vi "Tacking Helper - Waypoint Array Constructor.vi"(0 "Second Angle":dbl, 1 "Minimum Final Tack Distance (m?)":dbl, 2 "Starting\nArm Length":dbl, 3 "Second\nArm Length":dbl, 5 "Jump Length (m)":dbl, 7 "Starting Angle":dbl, 9 "Distance of each waypoint to boat":dbl[](array[numeric]), 12 "Array Beginning":i32, 13 "Waypoint Array In":T1[](array[typedef]), 14 "Boat Position":T3) -> (4 "Distance to boat":dbl, 6 "Final Index of\nWaypoint Array":i32, 8 "Intermediate \nWaypoint Array out":T1[](array[typedef]))   [LabVIEW 2011]
doc: "While the distance to the boat is greater than 1 jump (plus a minimum tack distance allowable we have yet to determine) the while loop will increment again and another two points will be calculated (one jump). The subvi inside of the loop takes the angles and lengths and actually adds the next step to the array.\n\nThe intermediate waypoint array output is the important thing - it stores each waypoint. The 'final index' and 'distance until boat' are used for plotting."
uses:
  2 Typedefs/UTM Location.ctl
  0x2-OCU-Think Comm/0x2 Typedefs/ocuWaypoint.ctl
  0x2-OCU-Think Comm/0x2 Typedefs/waypointTypes.ctl
  <vilib>/Analysis/_algsub.llb/Real Vector Norm.vi
  <vilib>/Analysis/NI_AALPro.lvlib
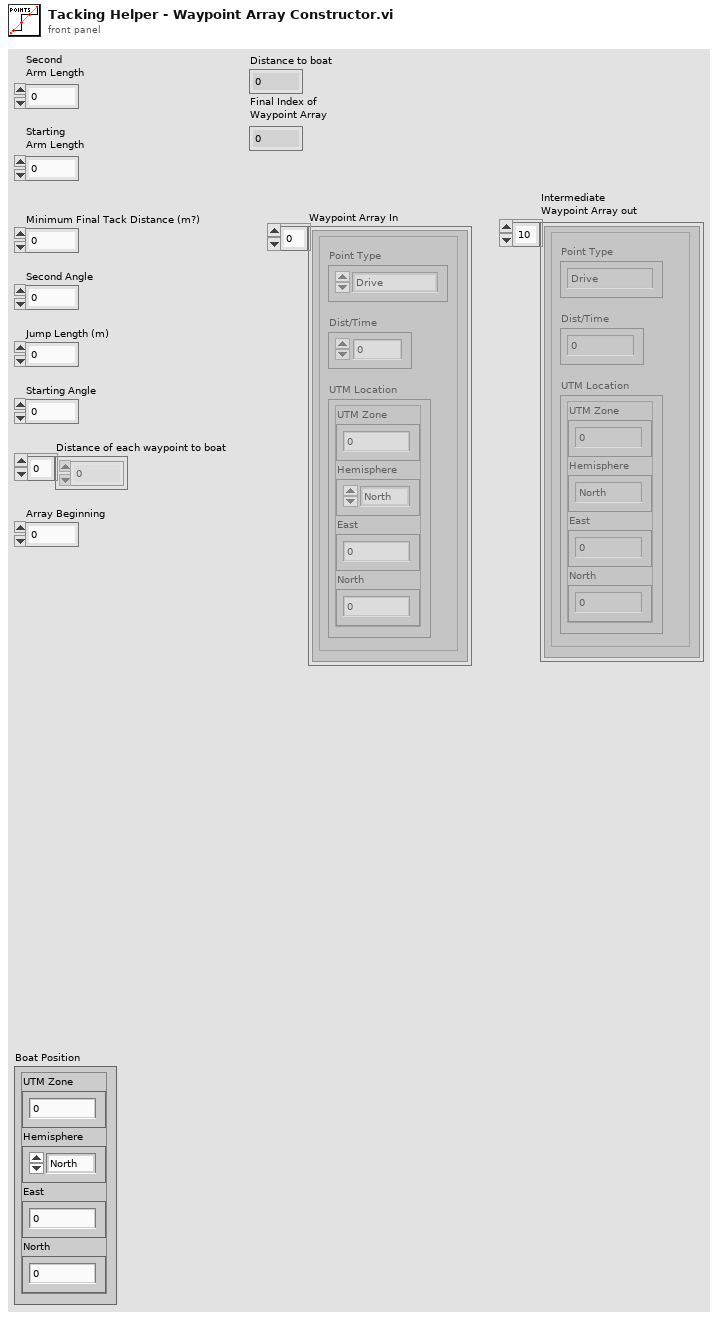
[diagram p1: front panel]
types:
  T1 = typedef "ocuWaypoint.ctl" = cluster{"Point Type":T2, "Dist/Time":dbl, "UTM Location":T3}
  T2 = typedef "waypointTypes.ctl" = enum16{"Drive", "Round Port", "Round Starboard", "Stay"}
  T3 = typedef "UTM Location.ctl" = cluster{"UTM Zone":dbl, "Hemisphere":enum16{"North", "South"}, "East":dbl, "North":dbl}
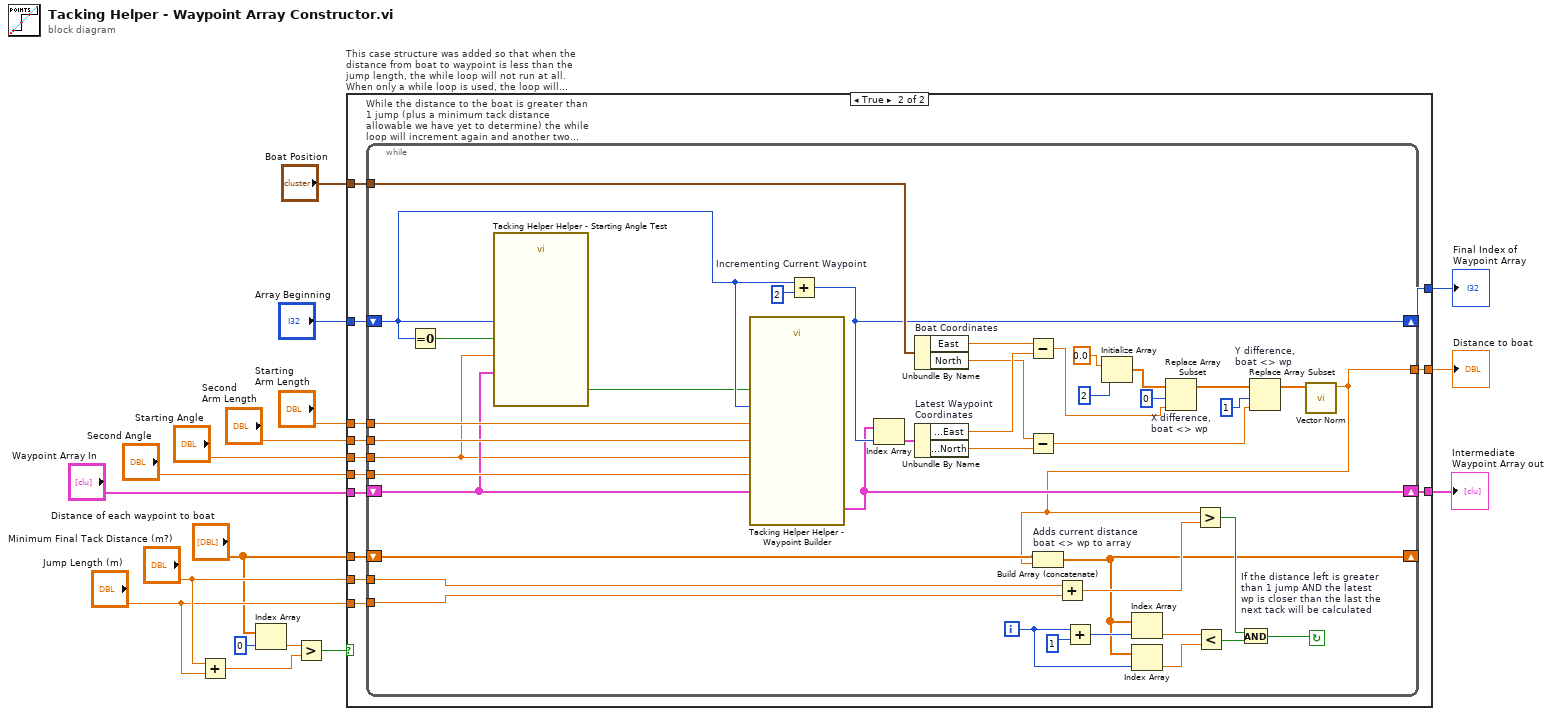
[diagram p0: block diagram]
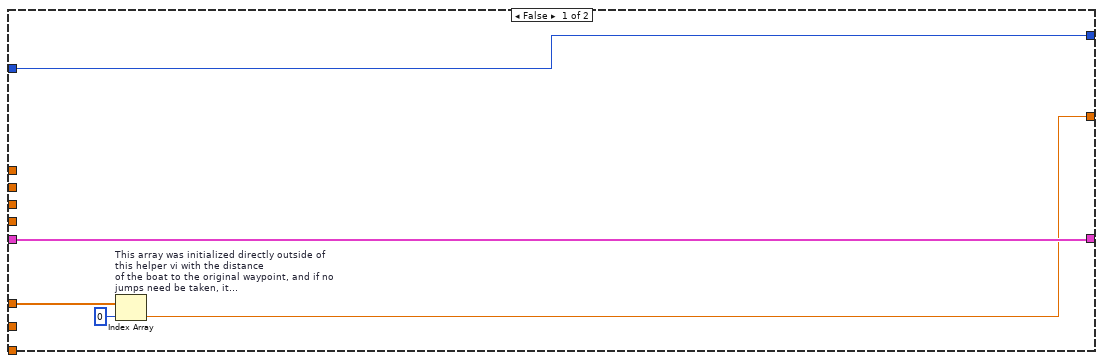
[diagram p2: hidden frame]
diagram:
  n1 = Add(x="Minimum Final Tack Distance (m?)", y="Jump Length (m)") -> (x+y=w6:dbl)
  n2 = Index Array(array="Distance of each waypoint to boat", index=0) -> (element=w1:dbl)
  n3 = Greater?(x=w1, y=w6) -> (0:w7:bool)
  n4 = case "This case structure was added so that when the distance from boat to waypoint is less than the jump length, the while loop will not run at all. When only a while loop is used, the loop will run\nonce no matter how close the boat is to the waypoint." shown="True" w7 {
    tunnel: "Minimum Final Tack Distance (m?)" -> [_ w35]
    tunnel: "Jump Length (m)" -> [_ w34]
    tunnel: "Starting Angle" -> [_ w33]
    tunnel: "Boat Position" -> [_ w32]
    tunnel: [w18 w31] -> w15
    tunnel: [w22 w30] -> w14
    tunnel: [w21 w29] -> w13
    tunnel: "Distance of each waypoint to boat" -> [w19 w28]
    tunnel: "Array Beginning" -> [w22 w27]
    tunnel: "Waypoint Array In" -> [w21 w26]
    tunnel: "Second Angle" -> [_ w25]
    tunnel: "Second\nArm Length" -> [_ w24]
    tunnel: "Starting\nArm Length" -> [_ w23]
    frame False {
      n5 = Index Array "This array was initialized directly outside of this helper vi with the distance\nof the boat to the original waypoint, and if no jumps need be taken, it\nshould simply pass that distance through"(array=w19, index=0) -> (element=w18:dbl)
    }
    frame True {
      n6 = while "While the distance to the boat is greater than 1 jump (plus a minimum tack distance allowable we have yet to determine) the while loop will increment again and another two points will be\ncalculated (one jump). The subvi inside of the loop actually takes the angles and lengths and actually adds the next step to the array.." {
        shift-right: [w71] -> w30
        shift-left: w27 -> [w39]
        shift-right: [w70] -> w29
        shift-left: w26 -> [w44]
        tunnel: w23 -> [w45]
        tunnel: w24 -> [w74]
        tunnel: w33 -> [w37]
        tunnel: w25 -> [w73]
        tunnel: w32 -> [w72]
        tunnel: w34 -> [w47]
        shift-right: [w38] -> _
        shift-left: w28 -> [w41]
        tunnel: [w40] -> w31
        tunnel: w35 -> [w48]
        i -> [w43]
        stop <- w53 continue-if-true
        n7 = Equal To 0?(x=w39) -> (x = 0?=w46:bool)
        n8 = call "Tacking Helper Helper - Starting Angle Test.vi"("Waypoint Array In"=w44, "Starting Angle"=w37, "Tests whether the while\nloop is on its first step"=w46, "Step Number\nof While Loop"=w39) -> ("Boolean out"=w36:bool)  [unwired: 7 in]
        n9 = call "Tacking Helper Helper - Waypoint Builder.vi"("Second Arm Length"=w74, "Current Waypoint\nBeing Adjusted"=w39, "Starting Arm Length"=w45, "Waypoint\nArray In"=w44, "Second Angle"=w73, "If true, the starting angle was\nthe last angle used, and will\nbe used first"=w36, "Starting Angle"=w37) -> ("Waypoint \nArray Out"=w70:T1[])  [unwired: 4 in]
        n10 = Add "Incrementing Current Waypoint"(x=w39, y=2) -> (x+y=w71:i32)
        n11 = Index Array(array=w70, index=w71) -> (element=w69:T1)
        n12 = Unbundle By Name "Boat Coordinates"(w72) -> ("East"=w68:dbl, "North"=w66:dbl)
        n13 = Unbundle By Name "Latest Waypoint\nCoordinates"(w69) -> ("UTM Location.East"=w67:dbl, "UTM Location.North"=w65:dbl)
        n14 = Subtract(x=w68, y=w67) -> (x-y=w60:dbl)
        n15 = Subtract(x=w66, y=w65) -> (x-y=w57:dbl)
        n16 = Add(x=w48, y=w47) -> (x+y=w55:dbl)
        n17 = Add(x=w43, y=1) -> (x+y=w49:i32)
        n18 = Initialize Array(0.0 ("element"), 2 ("dimension size")) -> (w62:dbl[])
        n19 = Replace Array Subset "X difference,\nboat <> wp"(array=w62, new element=w60, index=0) -> (w58:dbl[])
        n20 = Replace Array Subset "Y difference,\nboat <> wp"(array=w58, new element=w57, index=1) -> (w56:dbl[])
        n21 = call-poly <vilib>:"Vector Norm.vi"("Input Vector"=w56) -> ("norm"=w40:dbl)  [unwired: 9 in, 1 out]
        n22 = Build Array (concatenate) "Adds current distance\nboat <> wp to array"(w41, w40) -> (w38:dbl[])
        n23 = Index Array(array=w38, index=w49) -> (element=w52:dbl)
        n24 = Index Array(array=w38, index=w43) -> (element=w51:dbl)
        n25 = Greater?(x=w40, y=w55) -> (0:w54:bool)
        n26 = Less?(x=w52, y=w51) -> (x < y?=w42:bool)
        n27 = And "If the distance left is greater\nthan 1 jump AND the latest\nwp is closer than the last the\nnext tack will be calculated"(x=w54, y=w42) -> (x .and. y?=w53:bool)
      }
    }
  }
  "Distance to boat" <- w15
  "Final Index of\nWaypoint Array" <- w14
  "Intermediate \nWaypoint Array out" <- w13
